vi "OE2031&OE2041_Configure Sensitivity and Filter.vi"(7 "OE2041_Configure \nSens and Filter":T1={"Input Range"=0, "Sensitivity "=24, "Time Constant "=20, "Low Pass Filter Slope "=3, "Enable Sync Filter "=0} {"Enable Sync Filter" items=["OFF", "ON"]; "Low Pass Filter Slope" items=["6 dB/oct", "12 dB/oct", "18 db/oct", "24 dB/oct", "30 dB/oct", "36 dB/oct", "42 dB/oct", "48 dB/oct"]; "Time Constant" items=["30 ns", "60 ns", "125 ns", "250 ns", "500 ns", "1 us", "2 us", "4 us", "8 us", "16 us", "32 us", "64 us", "125 us", "250 us", "500 us", "1 ms", "2 ms", "4 ms", "8 ms", "16 ms", "32 ms", "65 ms", "125 ms", "250 ms", "500 ms", "1 s", "2 s", "4 s", "8 s", "17 s", "35 s", "70 s", "140 s", "275 s", "550 s", "1100 s", "2200 s", "4400 s"]; "Sensitivity" items=["1 nV/fA", "2 nV/fA", "5 nV/fA", "10 nV/fA", "20 nV/fA", "50 nV/fA", "100 nV/fA", "200 nV/fA", "500 nV/fA", "1 uV/pA", "2 uV/pA", "5 uV/pA", "10 uV/pA", "20 uV/pA", "50 uV/pA", "100 uV/pA", "200 uV/pA", "500 uV/pA", "1 mV/nA", "2 mV/nA", "5 mV/nA", "10 mV/nA", "20 mV/nA", "50 mV/nA", "100 mV/nA", "200 mV/nA", "500 mV/nA", "1 V/uA"]; "Input Range" items=["1V", "200mV", "50mV", "10mV", "2mV", "400uV"]}, 8 "Error in (no error)":errorcluster caption="error out（no error）", 9 "Remote Mode":u16(ring) items=["USB"=0, "RS232"=1, "Ethernet"=3], 10 "Connection ID in":refnum<k5>, 11 "VISA resource name":refnum<visa-resource-name>) -> (0 "Error out":errorcluster caption="error out", 1 "Output String":string, 2 "Connection ID out":refnum<k5>, 3 "VISA resource  out":refnum<visa-resource-name>)   [LabVIEW 2011]
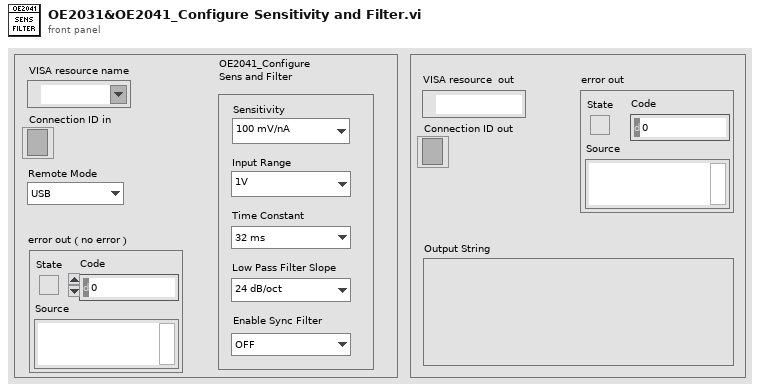
[diagram p1: front panel]
types:
  T1 = cluster{"Input Range":u16, "Sensitivity ":u16, "Time Constant ":u8, "Low Pass Filter Slope ":u8, "Enable Sync Filter ":u16}
  T2 = enum16{"ISRC", "IGND", "ICPL", "ILIN", "PHAS", "FMOD", "RSLP", "FREQ", "SWPT", "SLLM", "SULM", "SSLL", "SSLG", "STLM", "SWRM", "IRNG", "SENS", "RMOD", "OFLT", "OFSL", "SYNC", "DMOD", "HARM", "DARB", "SWVT", "SLVL", "SVLL", "SVUL", "SVSL", "SVSG", "SVTM", "SVRM", "RALL", "SNAP", "OUTP", "OAUX", "COUT", "CAUX", "COFP", "CEXP", "FPOP", "OEXP", "*IDN", "*RST", "OVLD", "INOV", "GNOV", "*PLL", "SSET", "RSET", "AGAN", "APHS", "ARSV", "ASCL", "EQCD", "EQCS", "SPED", "SRAT", "SLEN", "SSLE", "STRG", "SPRM", "STRD", "PAUS", "REST", "SPTS", "TRCA", "TEMP", "RSTU", "IHNZ", "DEQU", "SADD", "ARNG", "CSPE", "ISRCD", "IGNDD", "ICPLD", "ILIND", "PHASD", "FMODD", "RSLPD", "FREQD", "SWPTD", "SLLMD", "SULMD", "SSLLD", "SSLGD", "STLMD", "SWRMD", "SENSD", "RMODD", "OFLTD", "OFSLD", "SYNCD", "HARMD", "EQCDD", "EQCSD", "SNAPD", "OUTPD", "SWVTD", "SLVLD", "SVLLD", "SVULD", "SVSLD", "SVSGD", "SVTMD", "SVRMD", "SVDCD", "ARSVD", "AGAND", "APHSD", "ASCLD", "FPOPD", "CAUXD", "OEXPD", "SPEDD", "SRATD", "SLEND", "SSLED", "STRGD", "SPRMD", "STRDD", "PAUSD", "RESTD", "SPTSD", "TRCAD", "*IDND", "*RSTD", "INOVD", "GNOVD", "*PLLD", "SSETD", "RSETD"}
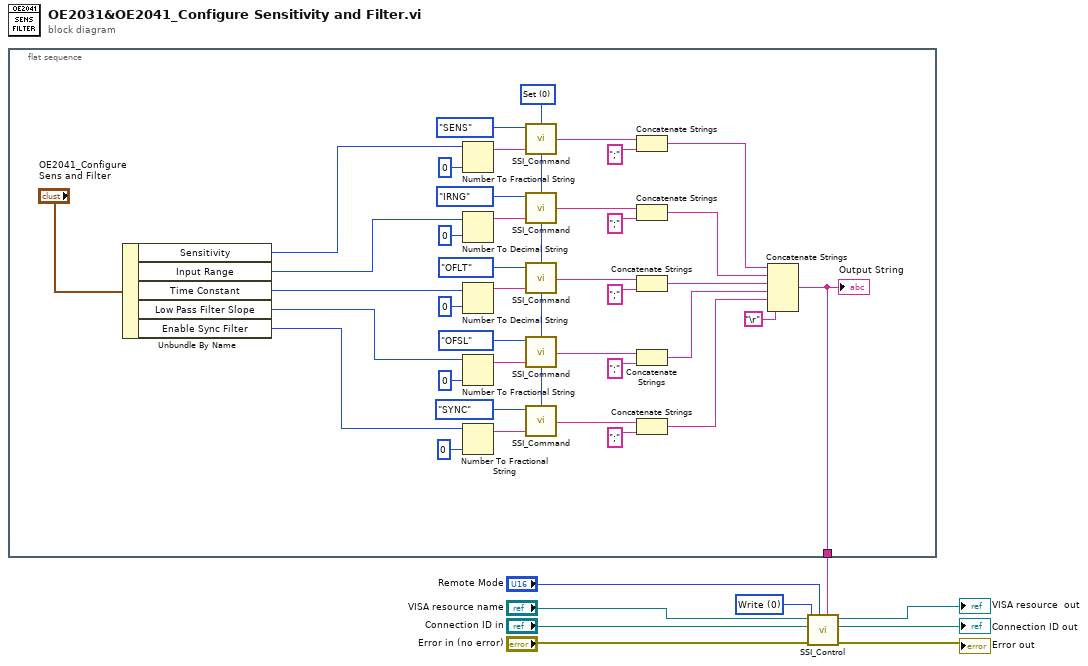
[diagram p0: block diagram]
diagram:
  w7 = u16 0 items=["Write", "Read"] ("Control")
  n1 = flat-sequence {
    tunnel: [w11] -> w1
    frame #0 {
      w19 = u16 0 items=["Set", "Query"] ("Opera")
      n2 = Unbundle By Name("OE2041_Configure \nSens and Filter") -> ("Sensitivity"=w29:u16, "Input Range"=w28:u16, "Time Constant"=w27:u8, "Low Pass Filter Slope"=w26:u8, "Enable Sync Filter"=w18:u16)
      n3 = Number To Fractional String(number=w29, precision (6)=i16 0 ("精度(6)")) -> (F-format string=w48:string)  [unwired: 2 in]
      n4 = Number To Decimal String(number=w28, width (-)=i16 0 ("宽度(-)")) -> (decimal integer string=w46:string)
      n5 = Number To Decimal String(number=w27, width (-)=i16 0 ("宽度(-)")) -> (decimal integer string=w44:string)
      n6 = Number To Fractional String(number=w26, precision (6)=i16 0 ("精度(6)")) -> (F-format string=w42:string)  [unwired: 2 in]
      n7 = Number To Fractional String(number=w18, precision (6)=i16 0 ("精度(6)")) -> (F-format string=w23:string)  [unwired: 2 in]
      n8 = call "SSI_Command.vi"("Opera"=w19, "Paramter"=w48, "Command Type"=T2."SENS") -> ("Output string"=w35:string)  [unwired: 1 in]
      n9 = call "SSI_Command.vi"("Opera"=w19, "Paramter"=w46, "Command Type"=T2."IRNG") -> ("Output string"=w39:string)  [unwired: 1 in]
      n10 = call "SSI_Command.vi"("Opera"=w19, "Paramter"=w44, "Command Type"=T2."OFLT") -> ("Output string"=w33:string)  [unwired: 1 in]
      n11 = call "SSI_Command.vi"("Opera"=w19, "Paramter"=w42, "Command Type"=T2."OFSL") -> ("Output string"=w37:string)  [unwired: 1 in]
      n12 = call "SSI_Command.vi"("Opera"=w19, "Paramter"=w23, "Command Type"=T2."SYNC") -> ("Output string"=w20:string)  [unwired: 1 in]
      n13 = Concatenate Strings(w35, ";" ("替换字符串(\"\")")) -> (w32:string)
      n14 = Concatenate Strings(w39, ";" ("替换字符串(\"\")")) -> (w31:string)
      n15 = Concatenate Strings(w33, ";" ("替换字符串(\"\")")) -> (w25:string)
      n16 = Concatenate Strings(w37, ";" ("替换字符串(\"\")")) -> (w24:string)
      n17 = Concatenate Strings(w20, ";" ("替换字符串(\"\")")) -> (w12:string)
      n18 = Concatenate Strings(w32, w31, w25, w24, w12, "\r") -> (w11:string)
      "Output String" <- w11
    }
  }
  n19 = call "SSI_Control.vi"("Write Buffer"=w1, "Remote Mode"="Remote Mode", "Error in (no error)"="Error in (no error)", "Control"=w7, "Connection ID in"="Connection ID in", "VISA resource name"="VISA resource name") -> ("Error out"=→"Error out":errorcluster, "Connection ID out"=→"Connection ID out":refnum<k5>, "VISA resource  out"=→"VISA resource  out":refnum<visa-resource-name>)  [unwired: 2 in, 1 out]
